vi "Read Path.vi"(8 "error in (no error)":errorcluster, 11 "Datalogger Path Set in":refnum<class "Datalogger Path Set Message.lvclass">) -> (0 "error out":errorcluster, 2 "Path":path, 3 "Datalogger Path Set out":refnum<class "Datalogger Path Set Message.lvclass">)   [LabVIEW 2018, in "Datalogger Path Set Message.lvclass"]
uses:
  Datalogger Path Set Message.lvclass
  Datalogger Path Set Message.lvclass/Datalogger Path Set Message.ctl
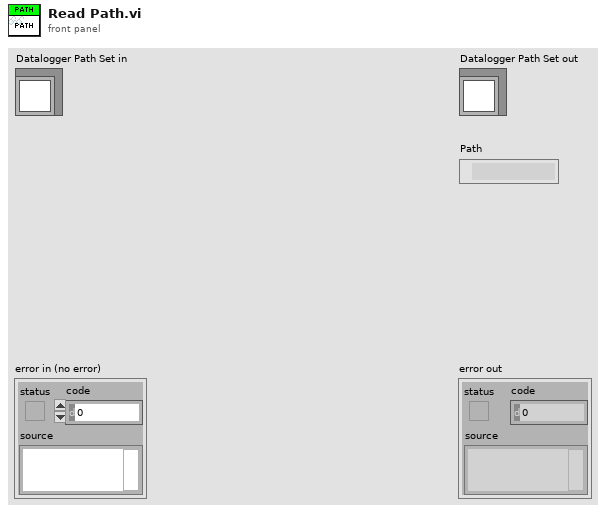
[diagram p1: front panel]
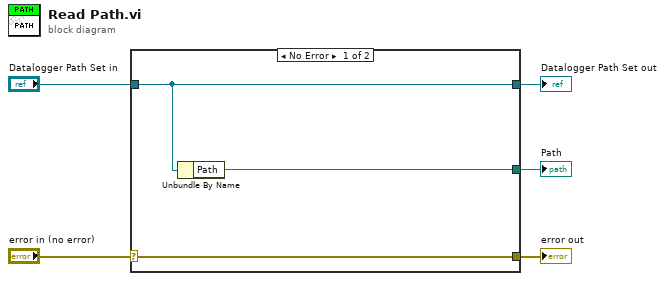
[diagram p0: block diagram]
diagram:
  n1 = case shown="No Error" "error in (no error)" {
    selector: "error in (no error)" -> [w8 w9]
    tunnel: [w8 w9] -> w4
    tunnel: [w7 w10] -> w2
    tunnel: "Datalogger Path Set in" -> [w7 w10]
    tunnel: [w6 _] -> w1
    frame No Error {
      n2 = Unbundle By Name(w7) -> ("Path"=w6:path)
    }
    frame Error {
    }
  }
  "error out" <- w4
  "Datalogger Path Set out" <- w2
  "Path" <- w1
